vi "DBL to Binary.vi"() -> ()   [LabVIEW 2016]
panel:
  out "DBL 3 Binary":bool[](array[boolean])
  in  "DBL 3":dbl
  out "DBL 2 Binary":bool[](array[boolean])
  in  "DBL 2":dbl
  in  "DBL 1":dbl
  out "DBL 1 Binary":bool[](array[boolean])
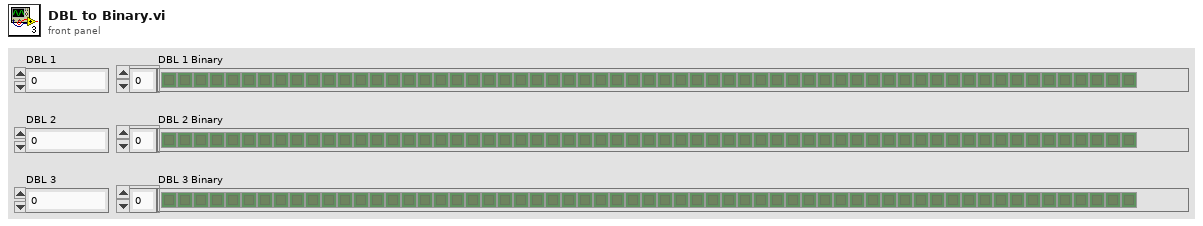
[diagram p1: front panel]
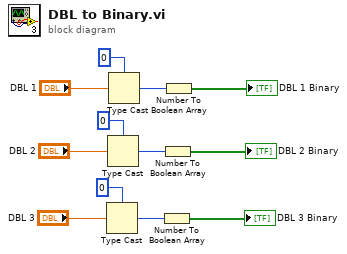
[diagram p0: block diagram]
diagram:
  n1 = Type Cast(type=u64 0, x="DBL 3") -> (*(type *) &x=w2:u64)
  n2 = Type Cast(type=u64 0, x="DBL 2") -> (*(type *) &x=w7:u64)
  n3 = Type Cast(type=u64 0, x="DBL 1") -> (*(type *) &x=w10:u64)
  n4 = Number To Boolean Array(number=w2) -> (Boolean array=→"DBL 3 Binary":bool[])
  n5 = Number To Boolean Array(number=w7) -> (Boolean array=→"DBL 2 Binary":bool[])
  n6 = Number To Boolean Array(number=w10) -> (Boolean array=→"DBL 1 Binary":bool[])
